vi "Second Derivative Matrices.vi"() -> (2 "d2/dx2":dbl[][](array[numeric])=[[0.0, 0.0, 0.0], [1.0, -2.0, 1.0], [0.0, 0.0, 0.0]], 3 "d2/dxdy":dbl[][](array[numeric])=[[1.0, 0.0, 1.0], [0.0, 0.0, 0.0], [-1.0, 0.0, -1.0]], 4 "d2/dy2":dbl[][](array[numeric])=[[0.0, 1.0, 0.0], [0.0, -2.0, 0.0], [0.0, 1.0, 0.0]], 5 "d":dbl[](array[numeric])=[-1.0, 0.0, 1.0])   [LabVIEW 2016]
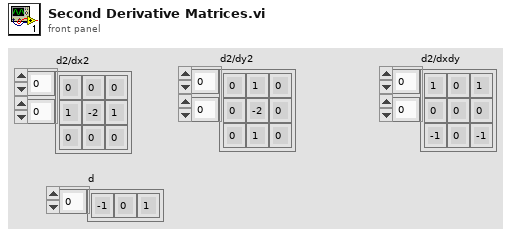
[diagram p1: front panel]
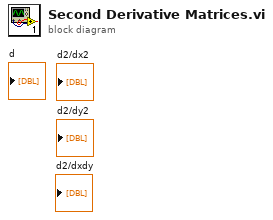
[diagram p0: block diagram]
diagram:
